vi "saveSetDirectory.vi"() -> (4 "pas":path, 6 "pd":path, 8 "processed":path, 10 "sweeps":path, 15 "crd":path)   [LabVIEW 2011]
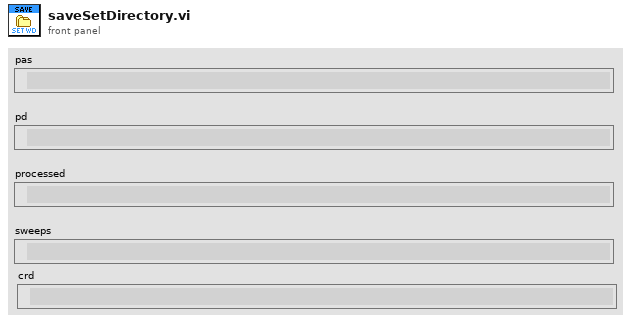
[diagram p1: front panel]
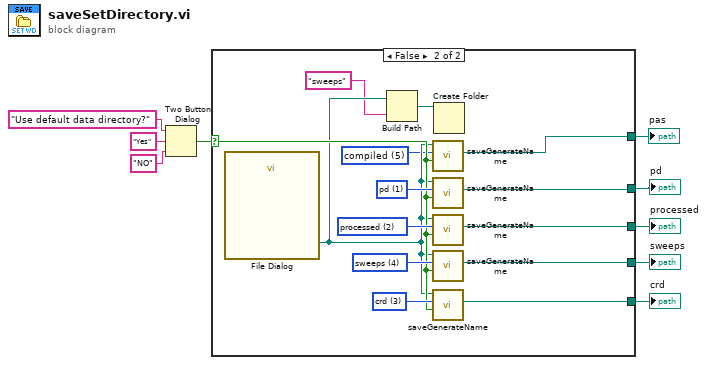
[diagram p0: block diagram]
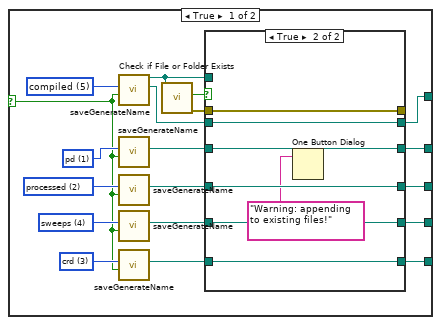
[diagram p2: hidden frame]
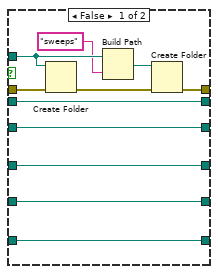
[diagram p3: hidden frame]
diagram:
  n1 = Two Button Dialog(message="Use default data directory?", 1:"NO" ("F button name (\"Cancel\")"), 2:"Yes" ("T button name (\"OK\")")) -> (T button?=w6:bool)
  n2 = case shown="False" w6 {
    selector: w6 -> [w24 w52]
    tunnel: [w19 w54] -> w7
    tunnel: [w17 w55] -> w8
    tunnel: [w15 w56] -> w9
    tunnel: [w12 w57] -> w1
    tunnel: [w21 w51] -> w2
    frame True {
      w10 = u16 5 items=["mic", "pd", "processed", "crd", "sweeps", "compiled"] ("Type")
      w25 = u16 3 items=["mic", "pd", "processed", "crd", "sweeps"] ("Type")
      w26 = u16 4 items=["mic", "pd", "processed", "crd", "sweeps"] ("Type")
      w27 = u16 2 items=["mic", "pd", "processed", "crd", "sweeps"] ("Type")
      w28 = u16 1 items=["mic", "pd", "processed", "crd", "sweeps"] ("Type")
      n3 = call "saveGenerateName.vi"("use default folder"=w24, "Type"=w10) -> ("file path"=w13:path, "working directory"=w11:path)  [unwired: 8 in]
      n4 = call "saveGenerateName.vi"("use default folder"=w24, "Type"=w28) -> ("file path"=w16:path)  [unwired: 8 in, 1 out]
      n5 = call "saveGenerateName.vi"("use default folder"=w24, "Type"=w27) -> ("file path"=w18:path)  [unwired: 8 in, 1 out]
      n6 = call "saveGenerateName.vi"("use default folder"=w24, "Type"=w26) -> ("file path"=w20:path)  [unwired: 8 in, 1 out]
      n7 = call "saveGenerateName.vi"("use default folder"=w24, "Type"=w25) -> ("file path"=w22:path)  [unwired: 8 in, 1 out]
      n8 = call <vilib>:"Check if File or Folder Exists.vi"("path"=w11) -> ("error out"=w14:errorcluster, "file or folder exists?"=w23:bool)  [unwired: 8 in, 1 out]
      n9 = case shown="True" w23 {
        tunnel: w22 -> [w36 w46]
        tunnel: [w36 w46] -> w21
        tunnel: w20 -> [w35 w45]
        tunnel: [w35 w45] -> w19
        tunnel: [w38 w44] -> w17
        tunnel: w18 -> [w38 w44]
        tunnel: w16 -> [w37 w43]
        tunnel: [w37 w43] -> w15
        tunnel: w14 -> [w39 w42]
        tunnel: [w29 w42] -> _
        tunnel: w13 -> [w34 w41]
        tunnel: [w34 w41] -> w12
        tunnel: w11 -> [w32 _]
        frame False {
          n10 = Create Folder(path (use dialog)=w32, error in=w39) -> (error out=w33:errorcluster)  [unwired: 1 in, 2 out]
          n11 = Build Path(base path=w32, name or relative path="sweeps") -> (appended path=w31:path)
          n12 = Create Folder(path (use dialog)=w31, error in=w33) -> (error out=w29:errorcluster)  [unwired: 1 in, 2 out]
        }
        frame True {
          n13 = One Button Dialog(message="Warning: appending to existing files!") -> ()  [unwired: 1 in, 1 out]
        }
      }
    }
    frame False {
      w47 = u16 5 items=["mic", "pd", "processed", "crd", "sweeps", "compiled"] ("Type")
      w53 = u16 3 items=["mic", "pd", "processed", "crd", "sweeps"] ("Type")
      w58 = u16 4 items=["mic", "pd", "processed", "crd", "sweeps"] ("Type")
      w59 = u16 2 items=["mic", "pd", "processed", "crd", "sweeps"] ("Type")
      w60 = u16 1 items=["mic", "pd", "processed", "crd", "sweeps"] ("Type")
      n14 = call "File Dialog"() -> ("selected path"=w50:path)  [unwired: 12 in, 3 out]
      n15 = Build Path(base path=w50, name or relative path="sweeps") -> (appended path=w49:path)
      n16 = call "saveGenerateName.vi"("use default folder"=w52, "Type"=w47, "working directory"=w50) -> ("file path"=w57:path)  [unwired: 7 in, 1 out]
      n17 = call "saveGenerateName.vi"("use default folder"=w52, "Type"=w60, "working directory"=w50) -> ("file path"=w56:path)  [unwired: 7 in, 1 out]
      n18 = call "saveGenerateName.vi"("use default folder"=w52, "Type"=w59, "working directory"=w50) -> ("file path"=w55:path)  [unwired: 7 in, 1 out]
      n19 = call "saveGenerateName.vi"("use default folder"=w52, "Type"=w58, "working directory"=w50) -> ("file path"=w54:path)  [unwired: 7 in, 1 out]
      n20 = call "saveGenerateName.vi"("use default folder"=w52, "Type"=w53, "working directory"=w50) -> ("file path"=w51:path)  [unwired: 7 in, 1 out]
      n21 = Create Folder(path (use dialog)=w49) -> ()  [unwired: 2 in, 3 out]
    }
  }
  "processed" <- w8
  "pd" <- w9
  "pas" <- w1
  "sweeps" <- w7
  "crd" <- w2
